vi "WriteChannel.vi"(8 "error in (no error)":errorcluster, 10 "Channel":i32, 11 "Television in":refnum<class "Television.lvclass">) -> (0 "error out":errorcluster, 3 "Television out":refnum<class "Television.lvclass">)   [LabVIEW 2013, in "Television.lvclass"]
uses:
  Television.lvclass
  Television.lvclass/Television.ctl
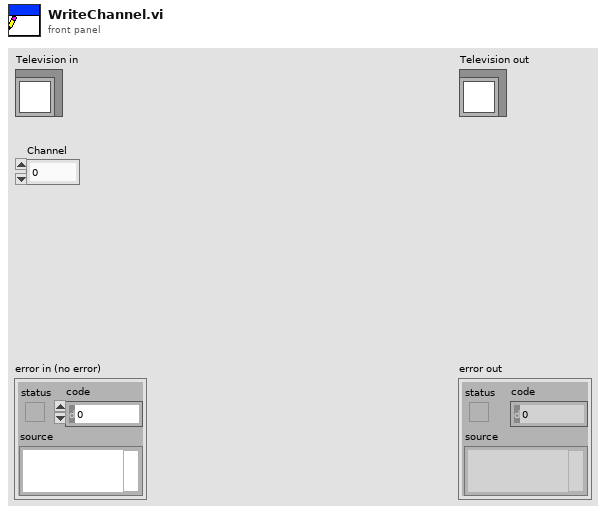
[diagram p1: front panel]
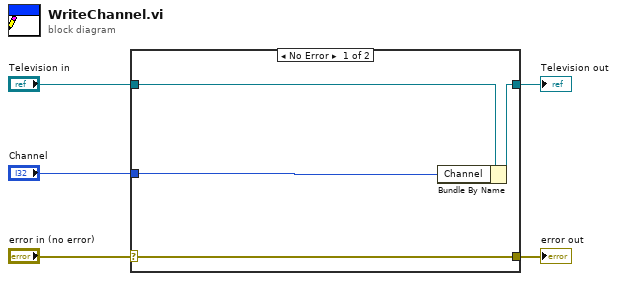
[diagram p0: block diagram]
diagram:
  n1 = case shown="No Error" "error in (no error)" {
    selector: "error in (no error)" -> [w9 w10]
    tunnel: [w9 w10] -> w4
    tunnel: [w7 w11] -> w2
    tunnel: "Television in" -> [w8 w11]
    tunnel: "Channel" -> [w6 _]
    frame No Error {
      n2 = Bundle By Name(cluster=w8, "Channel"=w6) -> (w7:refnum<class "Television.lvclass">)
    }
    frame Error {
    }
  }
  "error out" <- w4
  "Television out" <- w2
